vi "Read Module Menu Name.vi"(8 "error in":errorcluster, 11 "CVT editor node in":refnum<class "CVT editor node.lvclass">) -> (0 "error out":errorcluster, 2 "Menu Name":string, 3 "CVT editor node out":refnum<class "CVT editor node.lvclass">)   [LabVIEW 2013, in "CVT editor node.lvclass"]
uses:
  CVT editor node.lvclass
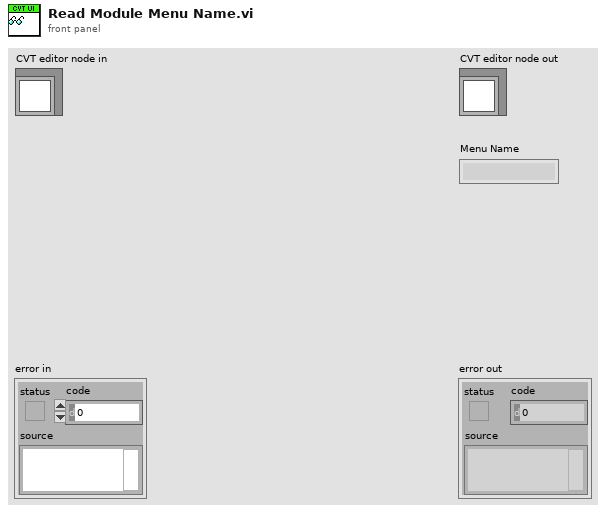
[diagram p1: front panel]
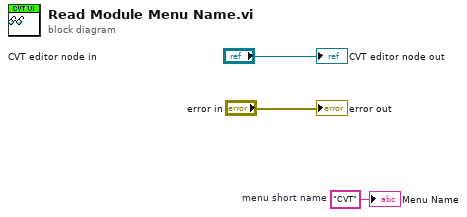
[diagram p0: block diagram]
diagram:
  w1 = "CVT"  # menu short name
  "error out" <- "error in"
  "CVT editor node out" <- "CVT editor node in"
  "Menu Name" <- w1
